vi "Channel Names and Default Values from Slot.vi"(8 "error in":errorcluster, 11 "slot ref in":T1 format="%.0x") -> (0 "error out":errorcluster, 1 "channel default values":dbl[](array[numeric]), 2 "channel names":string[](array[string]), 3 "slot ref out":T1 format="%.0x")   [LabVIEW 2017]
uses:
  <vilib>/NI Veristand/Custom Device API/Custom Device Item Ref.ctl
  <vilib>/NI Veristand/Custom Device Tools/Custom Device Utility Library/Custom Device Utility Library.lvlib
  <vilib>/NI Veristand/Custom Device API/Custom Device API.lvlib
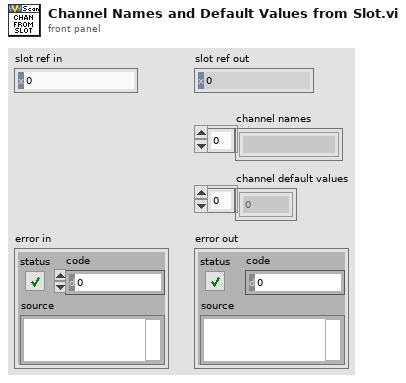
[diagram p1: front panel]
types:
  T1 = typedef "Custom Device API.lvlib/Custom Device Item Ref.ctl" = u64
  T2 = typedef "Custom Device API.lvlib/Custom Device Channel.ctl" = cluster{"Type":T3, "Units":string, "Default Value":dbl, "Faultable":bool, "Scalable":bool}
  T3 = typedef "Custom Device API.lvlib/Custom Device Channel Type.ctl" = enum16{"Input", "Output"}
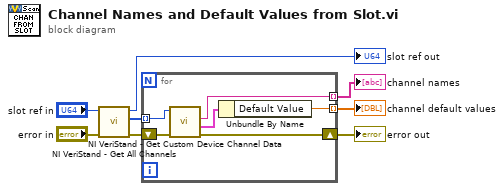
[diagram p0: block diagram]
diagram:
  n1 = call <vilib>:"NI VeriStand - Get All Channels.vi"("error in"="error in", "Section Ref in"="slot ref in") -> ("error out"=w4:errorcluster, "Channel Refs"=w3:T1[], "Section Ref out"=→"slot ref out":T1)  [unwired: 6 in, 1 out]
  n2 = for {
    tunnel: w3 -> [w13] mode=indexing
    shift-right: [w10] -> w6
    shift-left: w4 -> [w14]
    tunnel: [w12] -> w5 mode=indexing
    tunnel: [w9] -> w7 mode=indexing
    n3 = call <vilib>:"NI VeriStand - Get Custom Device Channel Data.vi"("error in (no error)"=w14, "Channel Ref in"=w13) -> ("error out"=w10:errorcluster, "Channel"=w11:T2, "Channel Name"=w12:string)  [unwired: 4 in, 3 out]
    n4 = Unbundle By Name(w11) -> ("Default Value"=w9:dbl)
  }
  "channel default values" <- w7
  "error out" <- w6
  "channel names" <- w5
